vi "templates preview template.vi"(6 "sxUsername":string, 8 "error in (no error)":errorcluster, 11 "sxTemplateID":string) -> (0 "error out":errorcluster, 3 "PNG":string)   [LabVIEW 2011]
uses:
  server/DIAdem/Datasheet/Datasheet Generator Settings.ctl
panel:
  in  "error.png":string
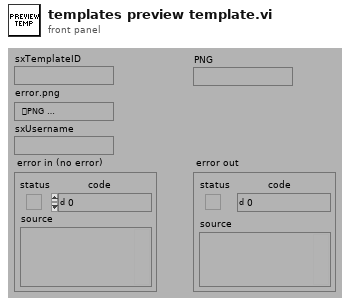
[diagram p1: front panel]
types:
  T1 = typedef "DATASHEET Generator Settings.ctl" = cluster{"Wait? (t)":bool, "ClientPrint? (f)":bool, "Client (\"\")":string, "joinPDF":bool, "Sort Method":enum16{"Item", "Template", "No Sort"}, "Export Row (-1=all)":i32, "Preview":bool, "Estimate Time":bool, "username":string, "jobid":string}
  T2 = typedef "Datasheet Report Info.ctl" = cluster{"sxTemplateId":string[], "reportPath":path}
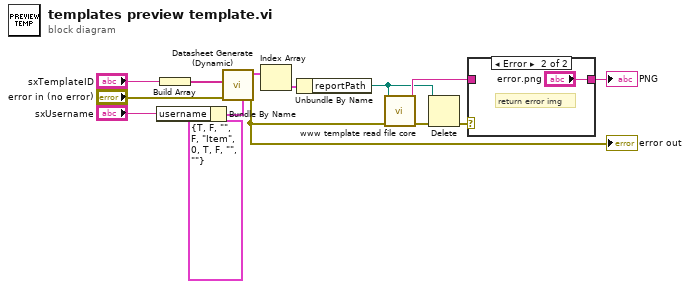
[diagram p0: block diagram]
diagram:
  n1 = Bundle By Name(cluster=T1 {"Wait? (t)"=TRUE, "ClientPrint? (f)"=FALSE, "Client (\"\")"="", "joinPDF"=FALSE, "Sort Method"=enum."Item", "Export Row (-1=all)"=0, "Preview"=TRUE, "Estimate Time"=FALSE, "username"="", "jobid"=""} ("Generator Settings"), "username"="sxUsername") -> (w3:T1)
  n2 = Build Array("sxTemplateID") -> (w5:string[])
  n3 = call "Datasheet Generate (Dynamic).vi"("Generator Settings"=w3, "error in (no error)"="error in (no error)", "Templates"=w5) -> ("error out"=w8:errorcluster, "Datasheet Paths"=w14:T2[])  [unwired: 6 in, 1 out]
  "error out" <- w8
  n4 = Index Array(array=w14) -> (element=w6:T2)  [unwired: 1 in]
  n5 = Unbundle By Name(w6) -> ("reportPath"=w2:path)
  n6 = call "www template read file core.vi"("error in (no error)"=w8, "Path"=w2) -> ("error out"=w12:errorcluster, "File Content"=w7:string)  [unwired: 8 out]
  n7 = Delete(path (use dialog)=w2, error in=w12) -> (error out=w11:errorcluster)  [unwired: 5 out]
  n8 = case shown="Error" w11 {
    tunnel: w7 -> [w15 _]
    tunnel: [w15 "error.png"] -> w13
    frame No Error {
    }
    frame Error {
      # "return error img"
    }
  }
  "PNG" <- w13
